vi "UI_page12.vi"(10 "传递队列输入":refnum<queue>, 11 "notifier":refnum<notifier>) -> ()   [LabVIEW 2012]
uses:
  <vilib>/Utility/miscctls.llb/LVDateTimeRec.ctl
  <vilib>/GPower/VIRegister/Library/Convert/ToBool.vi
  <vilib>/GPower/VIRegister/Library/Convert/ToU32.vi
  <vilib>/GPower/VIRegister/Library/Convert/ToU8.vi
  <vilib>/GPower/VIRegister/Library/SubVIs/FindRegisterData.vi
  <vilib>/GPower/VIRegister/Library/SubVIs/ReadSub.vi
  <vilib>/GPower/VIRegister/Library/SubVIs/WriteSub.vi
  <vilib>/GPower/Error/Library/FilterCodes.vi
  <vilib>/GPower/Error/Library/Filter/FilterMulti.vi
  <vilib>/GPower/VIRegister/Library/QManager/GetRegisterData.vi
  <vilib>/GPower/Error/Library/SetError.vi
  <vilib>/GPower/Error/Library/SplitAppended.vi
  <vilib>/GPower/VIRegister/Library/QManager/QManagerAction.vi
  <vilib>/GPower/Error/Library/ErrorType.vi
  <vilib>/GPower/Error/Library/SubVIs/ExplanationToError.vi
  <vilib>/GPower/VIRegister/Library/QManager/GetQName.vi
  <vilib>/GPower/VIRegister/Library/QManager/StartQManager.vi
  <vilib>/Utility/error.llb/Trim Whitespace.vi
  <vilib>/dlg_ctls.llb/Space Constant.vi
  <vilib>/Utility/error.llb/Error Code Database.vi
  <vilib>/GPower/Error/Library/SubVIs/SetStatus.vi
  <vilib>/GPower/Error/Library/AppendErrors.vi
  <vilib>/GPower/Error/Library/Append/AppendSingle.vi
  <vilib>/GPower/VIRegister/VIRegister.lvlib
  <vilib>/measure/NI_MABase.lvlib
panel:
  out "试验已用时":timestamp=timestamp(-28800 s since 1904-01-01) format="%<%H:%M:%S>T"
  in  "测试时间设定":timestamp=timestamp(-28800 s since 1904-01-01) format="%<%H:%M:%S>T"
  in  "停止测量":bool
  in  "开始测量":bool
  out "温度":string
  out "脉冲计数":string
  out "主份G3陀螺脉冲计数":dbl(graph)
  out "主份A3加速度计脉冲计数":dbl(graph)
  out "主份G2陀螺脉冲数":dbl(graph)
  out "主份A2加速度计脉冲计数":dbl(graph)
  out "主份G1陀螺脉冲数":dbl(graph)
  out "主份A1加速度计脉冲计数":dbl(graph)
  out "正确帧计数":u16
  out "错误帧计数":u32
  in  "加计大小量程":enum32{"小量程", "大量程"}(radio)=enum."大量程"
  in  "穿插错误":bool
  in  "少数据字":bool
  in  "少验和":bool
  in  "少帧头":bool
  in  "验和错":bool
  in  "帧头错":bool
  in  "无数据":bool
  in  "地检按钮":bool
  in  "加表频率":dbl=1.0 min=0.1 max=10.0 step=0.1
  in  "加表幅值":dbl=1.0
  in  "陀螺频率":dbl=1.0 min=0.1 max=10.0 step=0.1
  in  "陀螺幅值":dbl=1.0
  # "主  份"
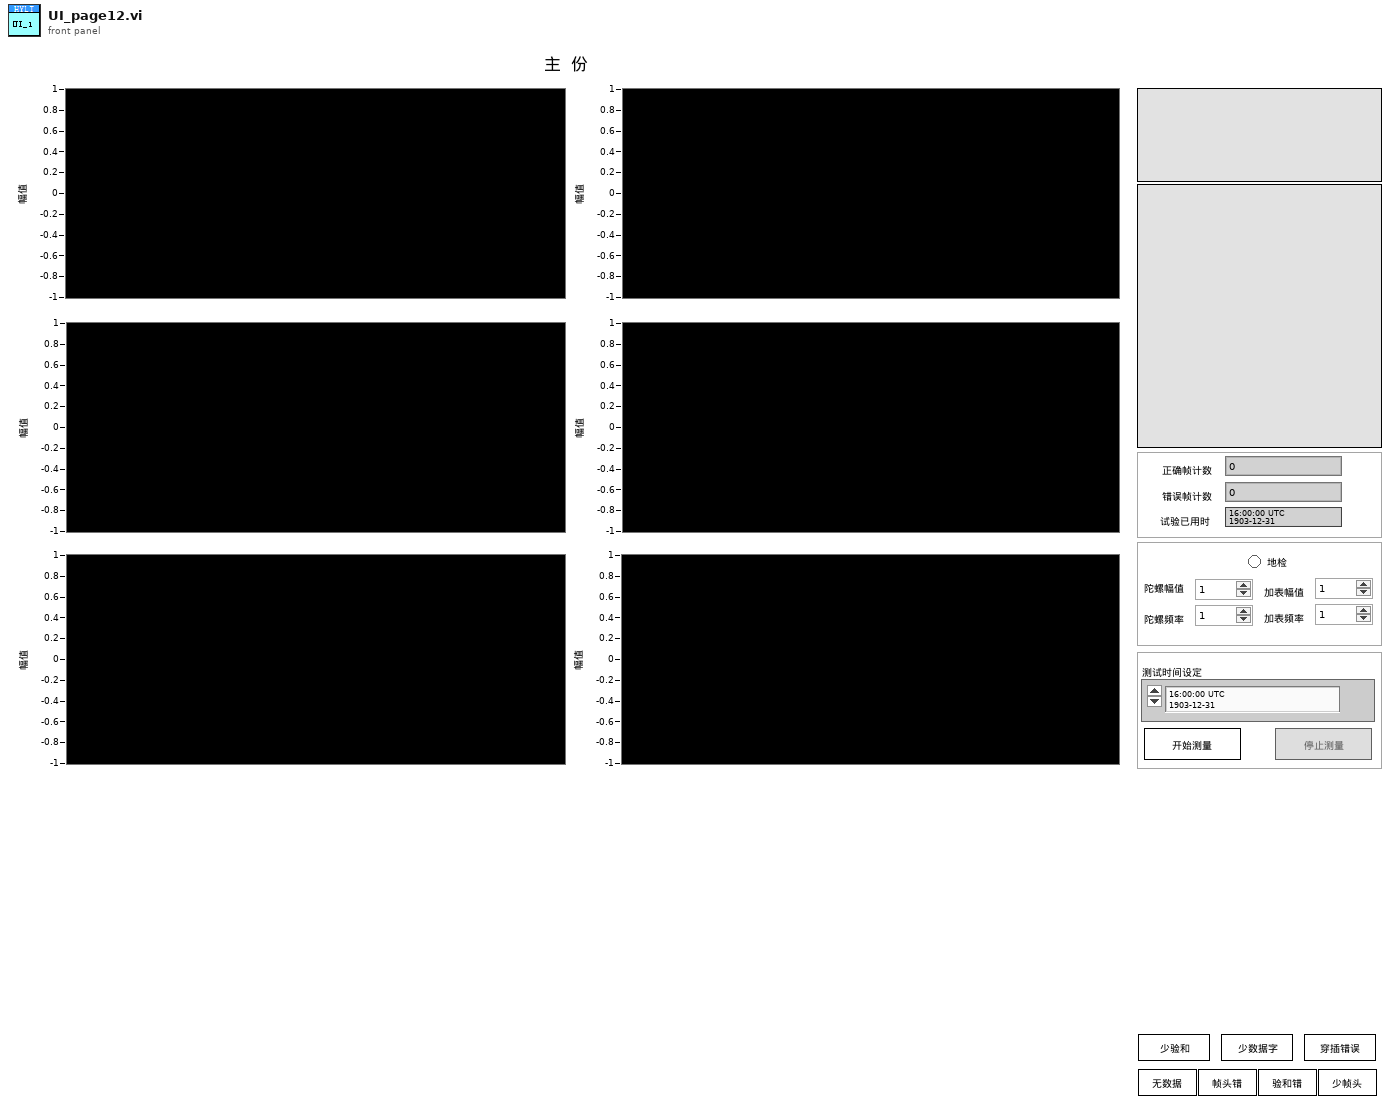
[diagram p1: front panel]
types:
  T1 = typedef "LVDateTimeRec.ctl" = cluster{"fractional second":dbl, "second":i32, "minute":i32, "hour":i32, "day of month":i32, "month":i32, "year":i32, "day of week":i32, "day of year":i32, "DST":i32}
  T2 = enum8{"Enabled", "Disabled", "Disabled and Grayed Out"}
  T3 = enum32{"invalid app kind", "Development System", "Run Time System", "Student Edition", "Embedded LabVIEW", "Evaluation", "Custom"}
  T4 = enum32{"Invalid", "Standard", "Closed", "Hidden", "Minimized", "Maximized"}
  T5 = cluster{"Core":cluster{"Current VI Reference":refnum<vi>, "Close Panel on Exit?":bool}, "传递队列输入":refnum<queue>, "信息帧":cluster{" 数据帧名称":string, " 数据":string, "备用操作符":bool, "起始地址":i32, "读写标志":i32, "长度":i32}, "主份控制指令":u16, "备份控制指令":u16, "notifier ":refnum<notifier>, "秒计数":i64, "起始时间":i64, "定时控制":bool}
  T6 = cluster{" 数据帧名称":string, " 数据":string, "备用操作符":bool, "起始地址":i32, "读写标志":i32, "长度":i32}
  T7 = cluster{"Current VI Reference":refnum<vi>, "Close Panel on Exit?":bool}
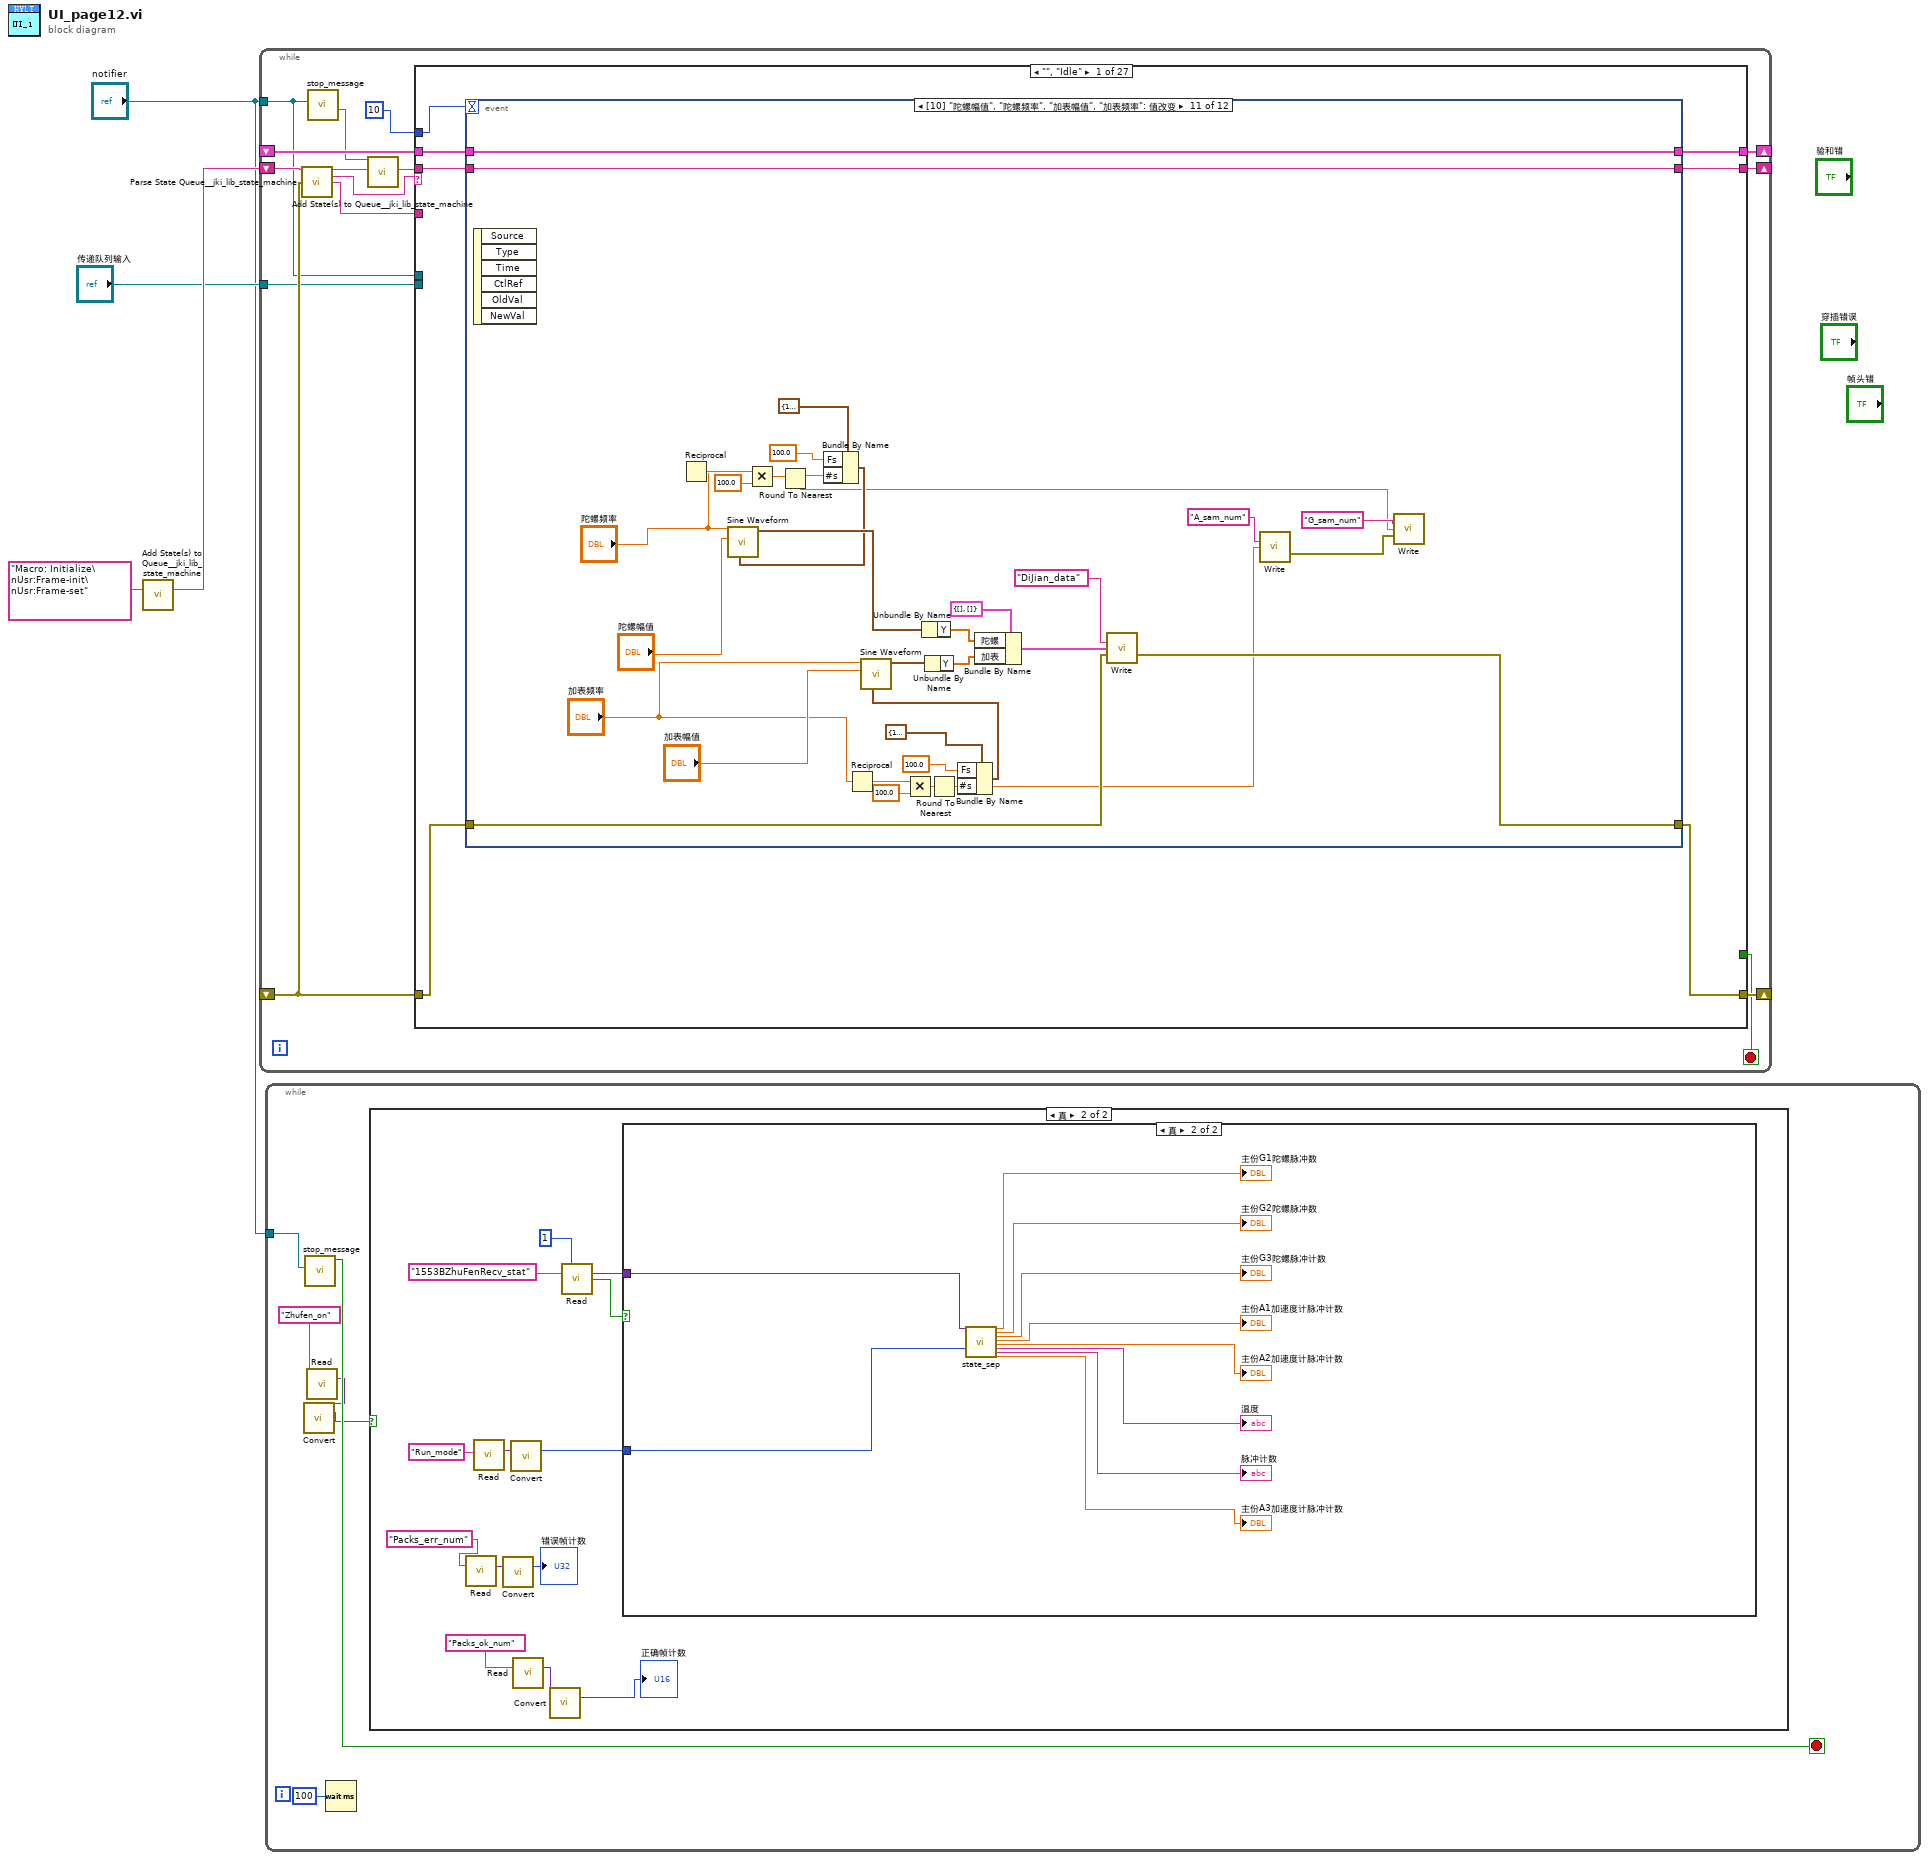
[diagram p0: block diagram]
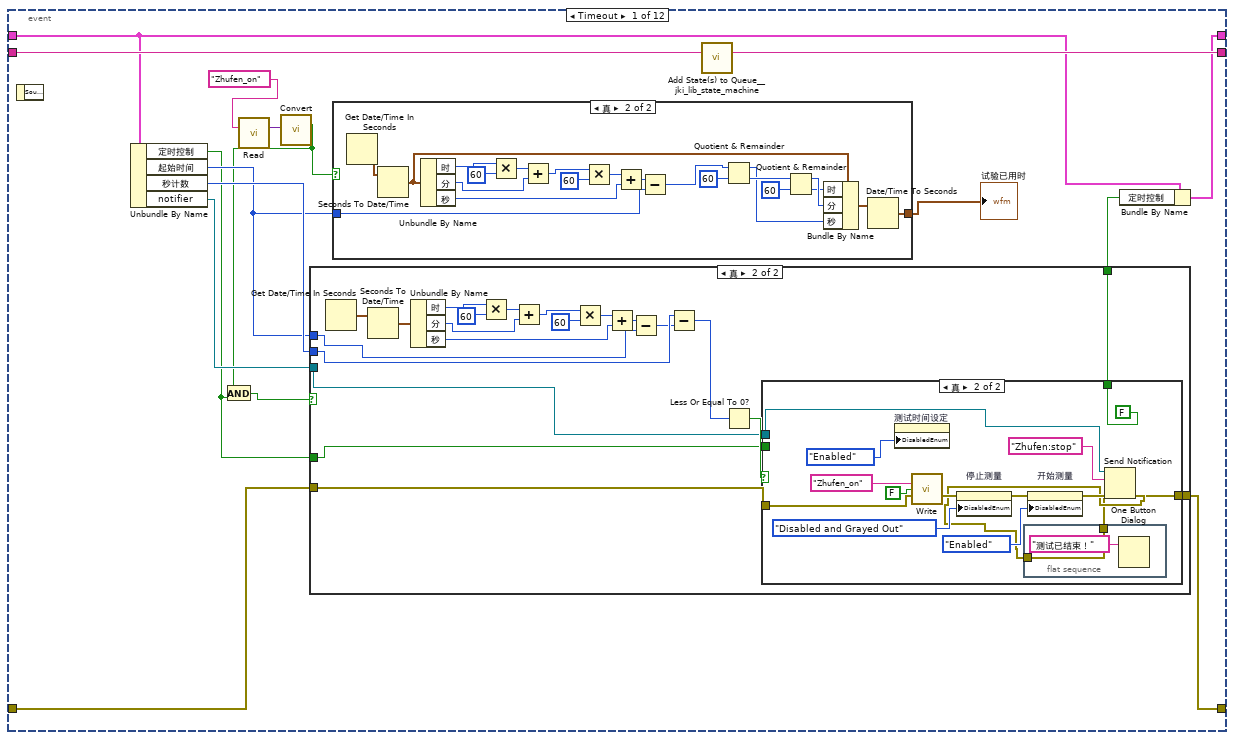
[diagram p4: hidden frame]
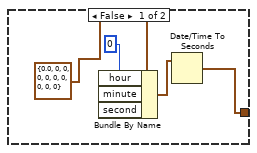
[diagram p5: hidden frame]
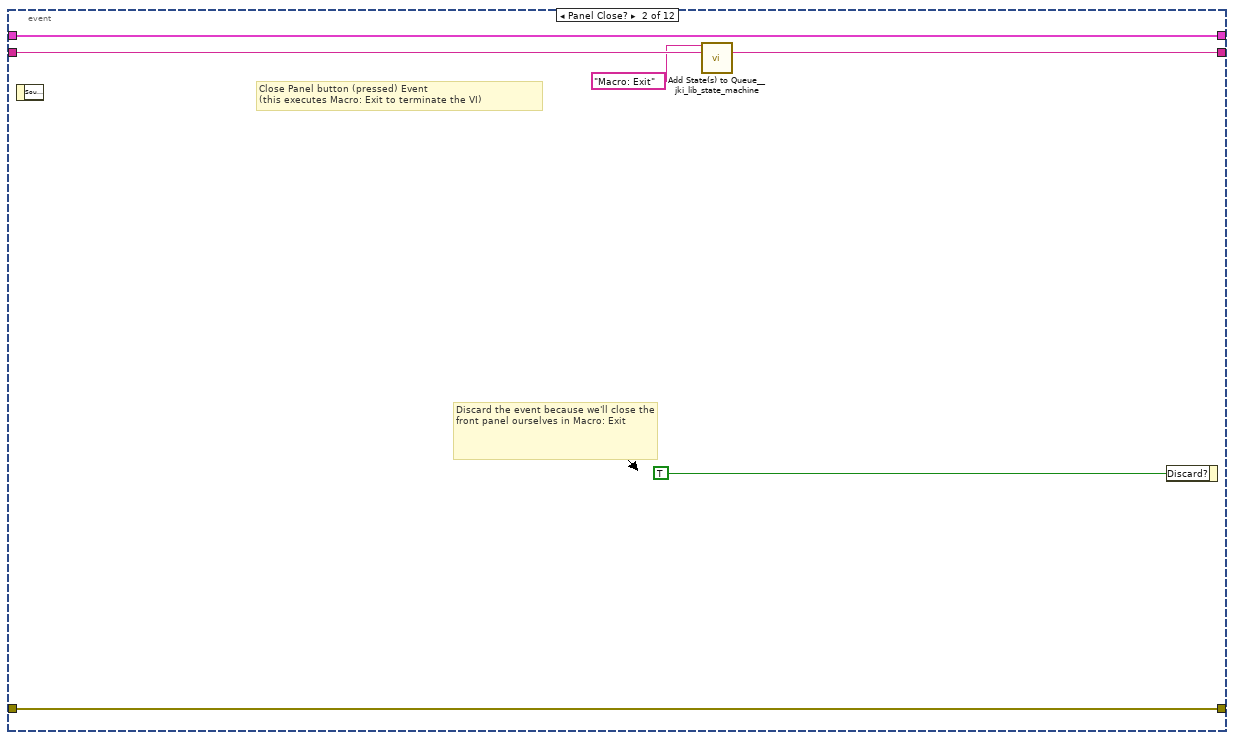
[diagram p8: hidden frame]
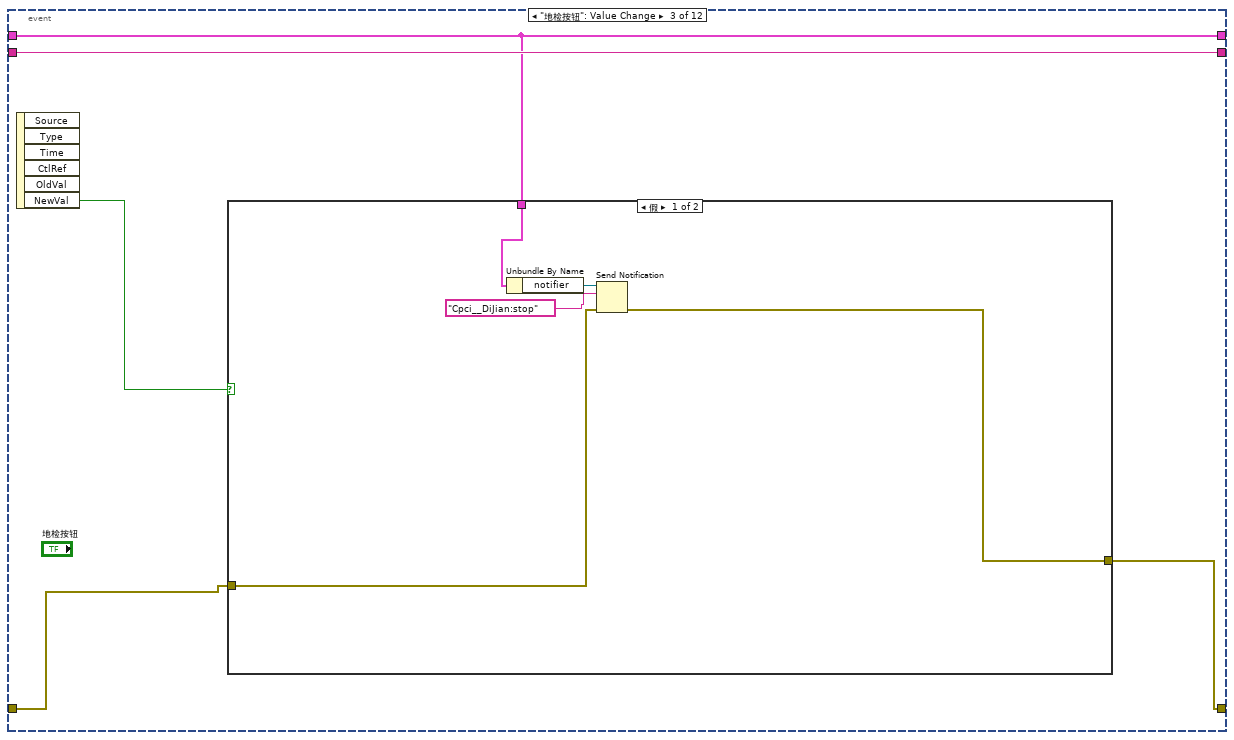
[diagram p9: hidden frame]
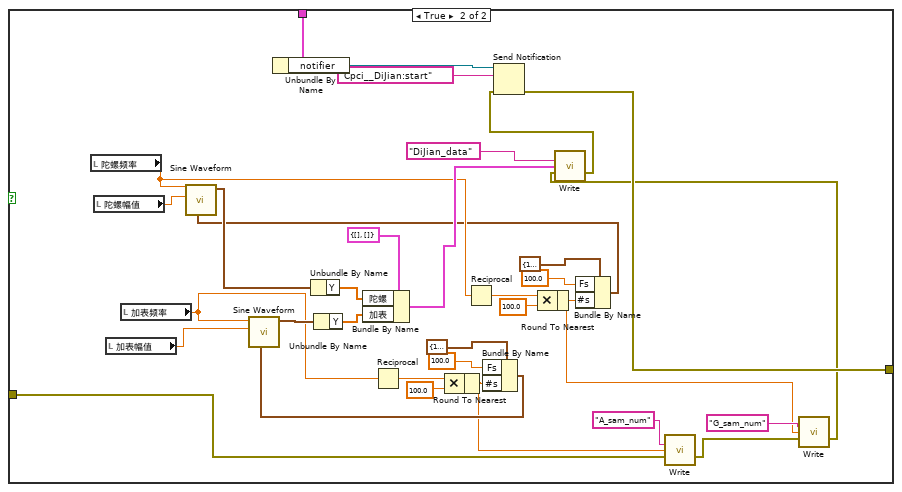
[diagram p10: hidden frame]
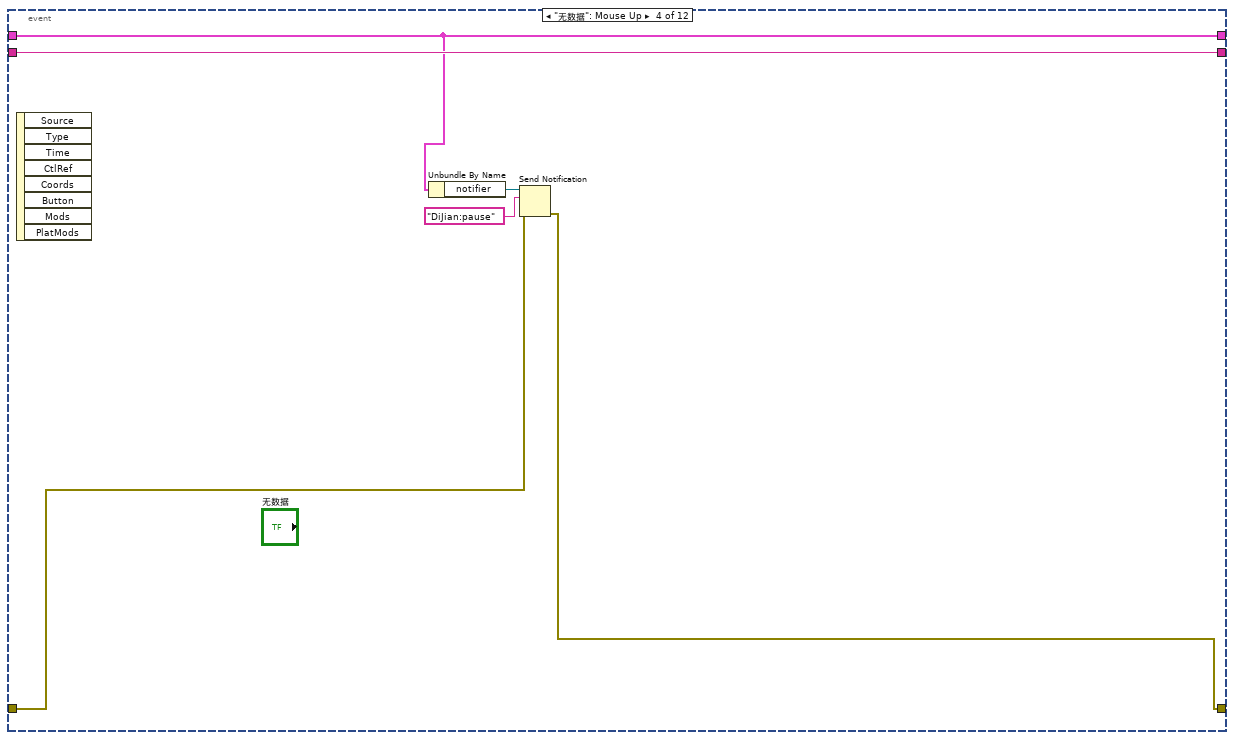
[diagram p11: hidden frame]
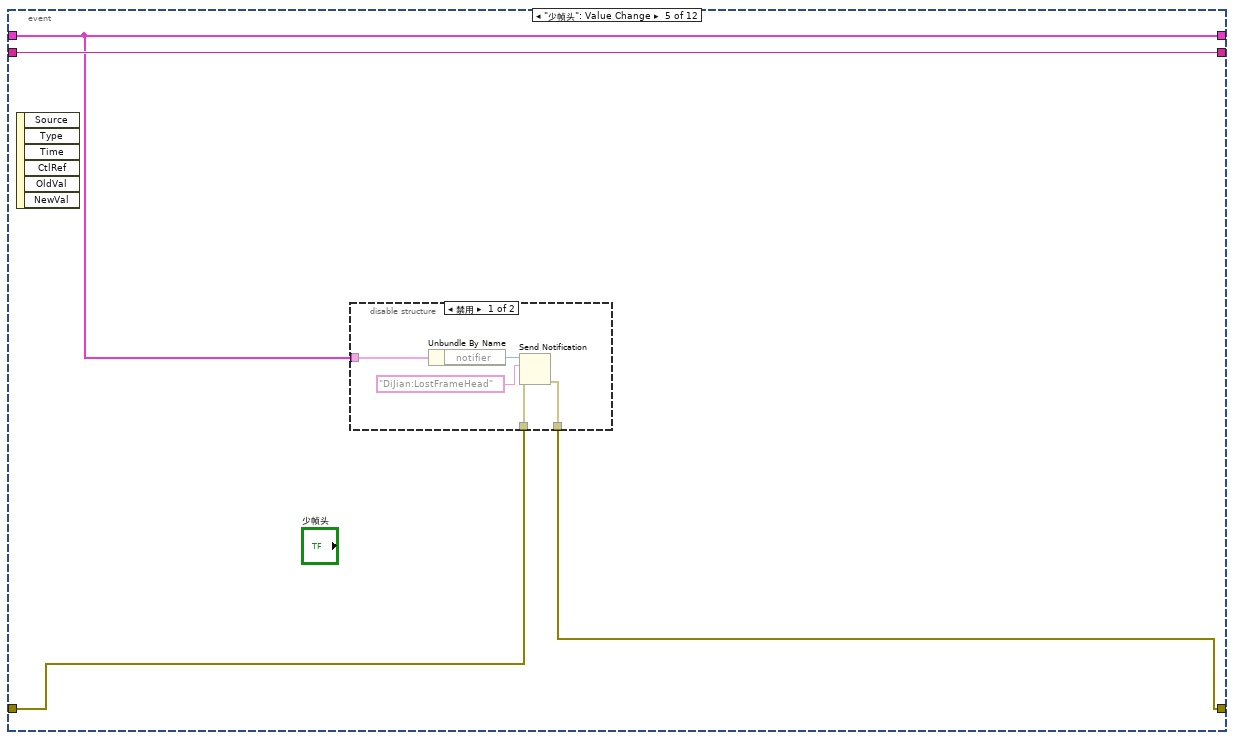
[diagram p12: hidden frame]
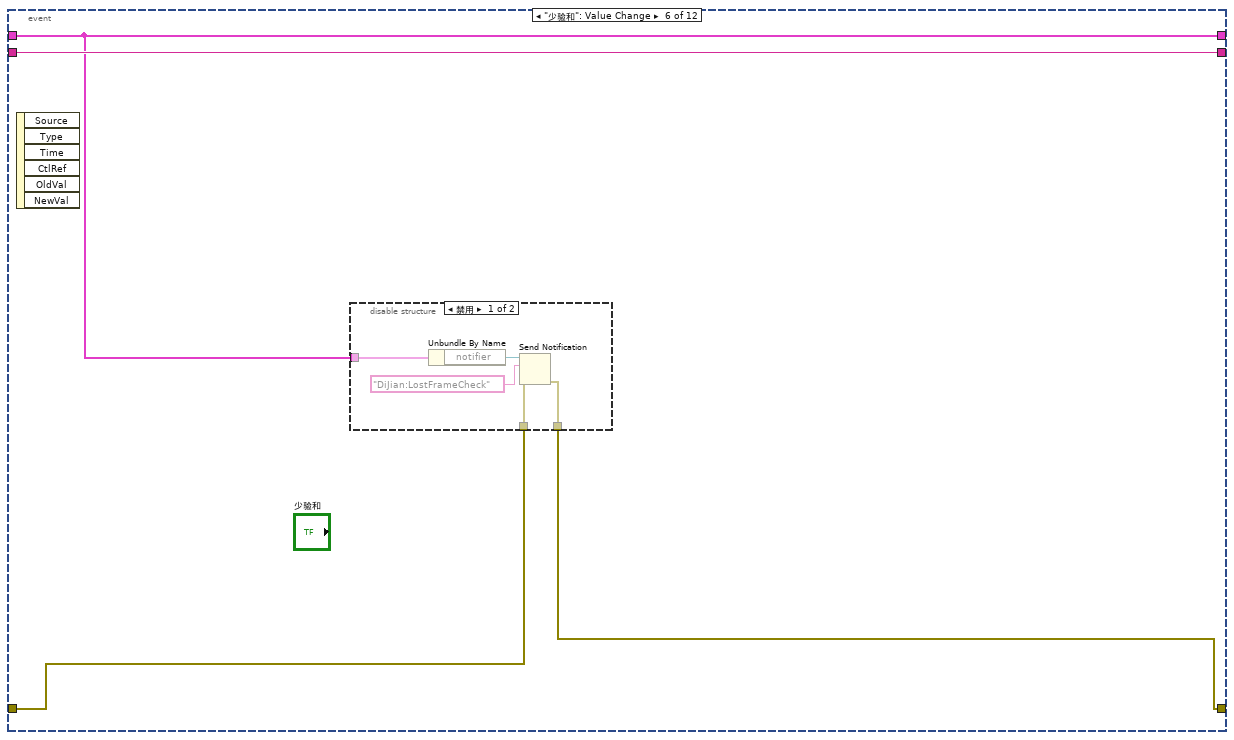
[diagram p14: hidden frame]
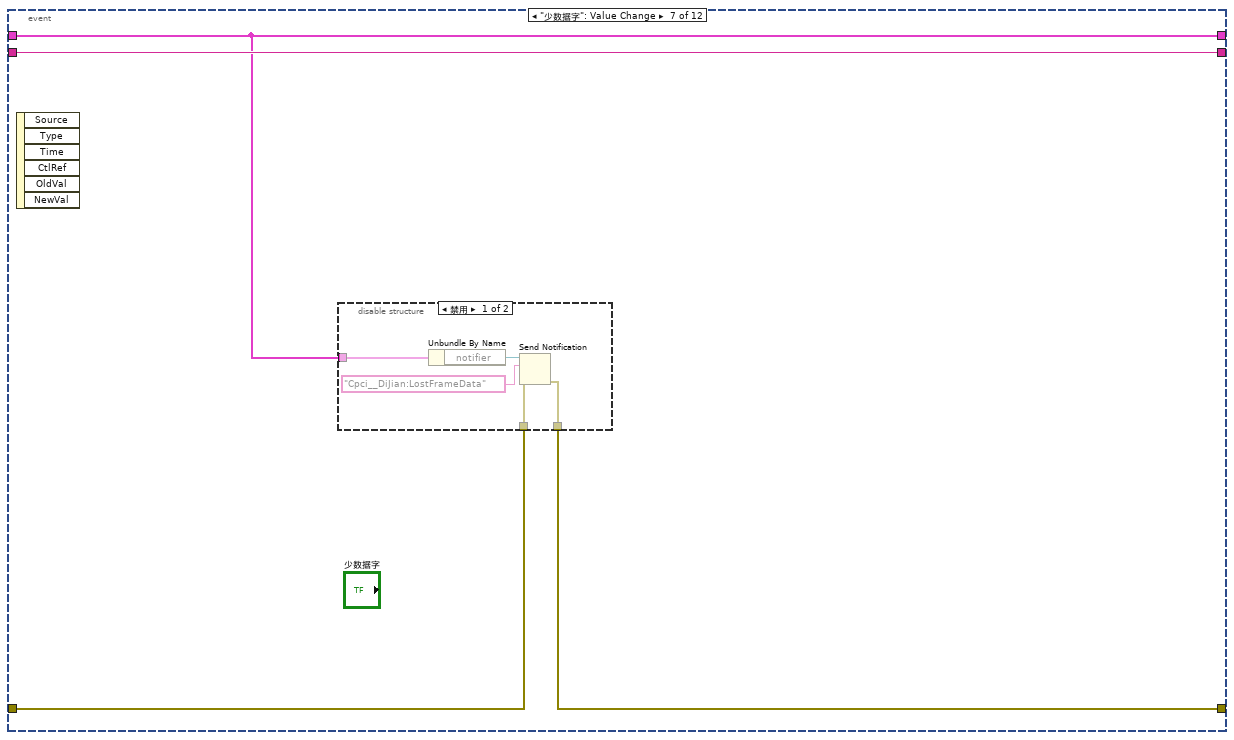
[diagram p16: hidden frame]
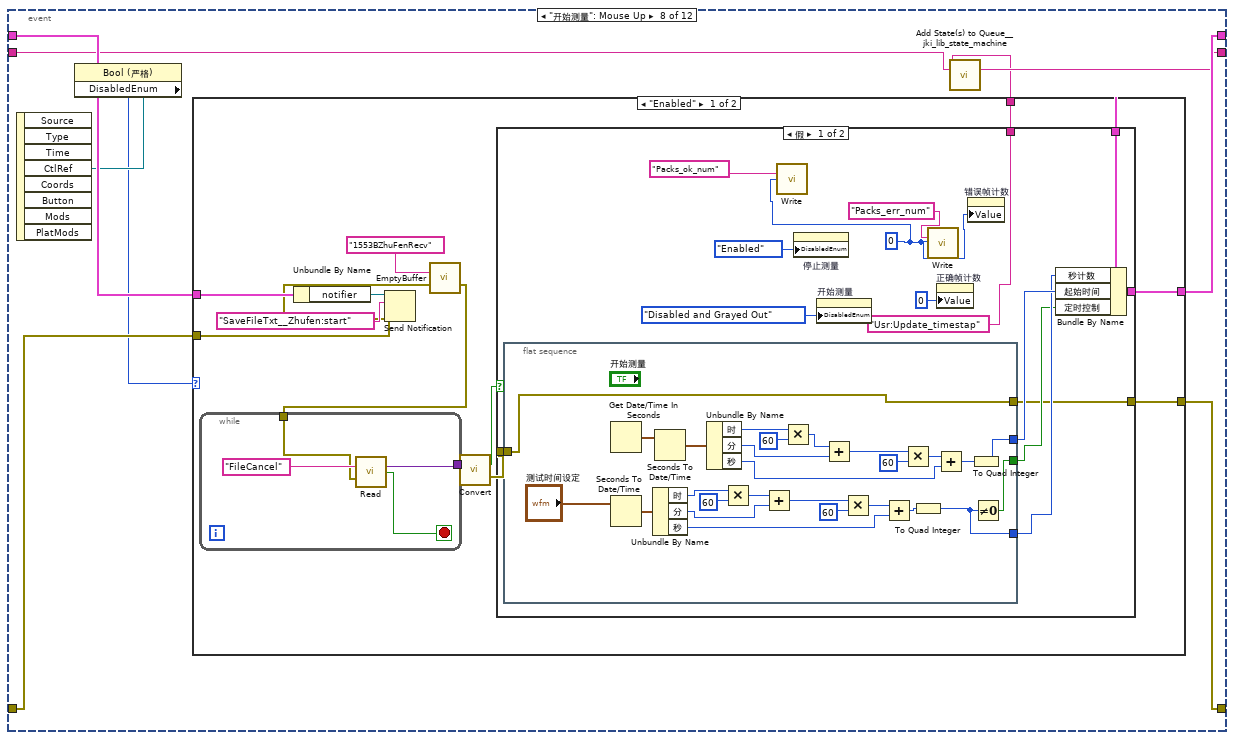
[diagram p18: hidden frame]
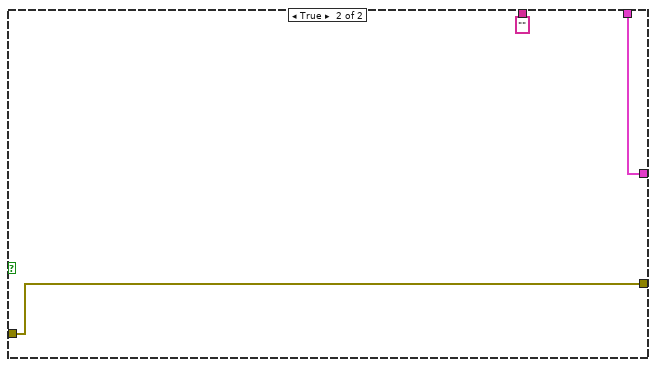
[diagram p19: hidden frame]
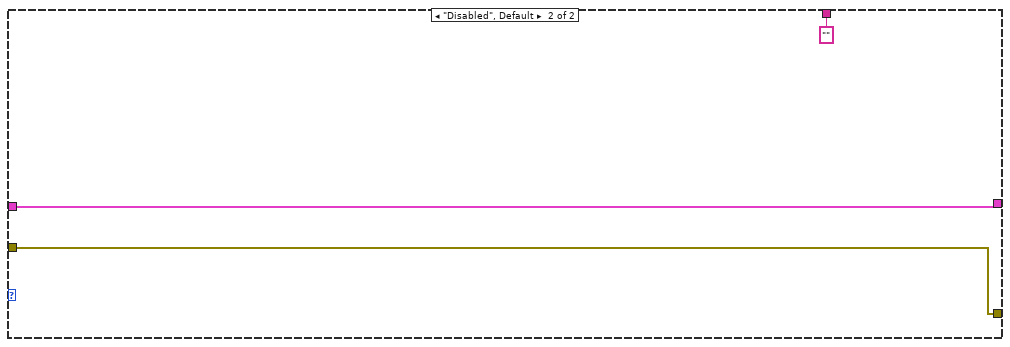
[diagram p20: hidden frame]
diagram:
  n1 = call <vilib>:"Add State(s) to Queue__jki_lib_state_machine.vi"("State(s) in (\"\")"="Macro: Initialize\nUsr:Frame-init\nUsr:Frame-set") -> ("States Out"=w4:string)  [unwired: 14 in]
  n2 = while "JKI - String-Based Queued State Machine (Basic) v1.0" {
    shift-right: [w13] -> _
    shift-left: _ -> [w12]
    shift-right: [w16] -> _
    shift-left: _ -> [w10]
    shift-right: [w15] -> _
    shift-left: w4 -> [w17]
    tunnel: "notifier" -> [w5]
    tunnel: "传递队列输入" -> [w6]
    stop <- w14 stop-if-true
    n3 = call <vilib>:"Parse State Queue__jki_lib_state_machine.vi"("State Queue"=w17, "Error In (no error)"=w10) -> ("Remaining States"=w9:string, "Current State"=w19:string, "Arguments"=w18:string)  [unwired: 11 in]
    n4 = call "stop_message.vi"("notifier"=w5) -> ("通知"=w8:string)  [unwired: 9 in, 1 out]
    n5 = call <vilib>:"Add State(s) to Queue__jki_lib_state_machine.vi"("State(s) in Front (\"\")"=w8, "State(s) in (\"\")"=w9) -> ("States Out"=w7:string)  [unwired: 13 in]
    n6 = case shown="\"\", \"Idle\"" w19 {
      selector: w19 -> [_ _ w352 _ _ _ _ _ _ _ _ _ _ _ _ _ _ _ _ _ _ _ _ _ _ _ _]
      tunnel: w7 -> [w20 w351 w356 w374 w380 w385 w389 w405 w411 w415 w424 w430 w440 w472 w477 w487 w491 w498 w518 w538 w557 w583 w599 w604 w609 w621 w639]
      tunnel: w18 -> [_ _ _ _ _ _ _ _ _ _ _ w425 w435 _ _ _ _ w492 w512 w532 _ _ _ _ _ _ _]
      tunnel: w12 -> [w25 w348 w354 w365 w377 w383 w386 _ w406 w412 w422 w428 w436 w469 w474 w484 w488 w496 w516 w536 w555 w581 w596 w601 w606 w617 w626]
      tunnel: [w24 w349 w358 w371 errorcluster {"status"=FALSE, "code"=0, "source"=""} ("error out") w382 w387 w402 w407 w413 w421 w426 w437 w470 w475 w485 w489 w494 w514 w534 w553 w579 w597 w602 w607 w619 w624] -> w16
      tunnel: w10 -> [w23 w349 w357 w371 w376 w382 w387 w402 w408 w413 w421 w427 w438 w470 w475 w485 w489 w495 w515 w535 w554 w580 w597 w602 w607 w619 w624]
      tunnel: [w26 w350 w355 w373 w379 w384 w388 w404 w410 w414 w423 w429 w439 w471 w476 w486 w490 w497 w517 w537 w556 w582 w598 w603 w608 w620 w638] -> w15
      tunnel: [_ _ _ _ _ TRUE _ _ _ _ _ _ _ _ _ _ _ _ _ _ _ _ _ _ _ _ _] -> w14
      tunnel: [w22 w348 w354 w372 w377 w383 w386 w403 w406 w412 w422 w428 w436 w469 w474 w484 w488 w493 w513 w533 w552 w578 w596 w601 w605 w617 w625] -> w13
      tunnel: 10 ("Timeout") -> [w21 _ _ _ _ _ _ _ _ _ _ _ _ _ _ _ _ _ _ _ _ _ _ _ _ _ _]
      tunnel: w6 -> [_ _ _ _ _ _ _ w399 _ _ _ _ _ _ _ _ _ _ _ _ _ _ _ _ _ _ _]
      tunnel: w5 -> [_ _ _ _ _ _ _ w395 _ _ _ _ _ _ _ _ _ _ _ _ _ _ _ _ _ _ _]
      frame "", "Idle" {
        n7 = event shown="[10] \"陀螺幅值\", \"陀螺频率\", \"加表幅值\", \"加表频率\": 值改变" {
          selector: _ -> [_ _ _ _ _ _ _ _ _ _ _ _]
          dyn-events: _ -> [_ _ _ _ _ _ _ _ _ _ _ _]
          timeout: w21 -> [_ _ _ _ _ _ _ _ _ _ _ _]
          tunnel: w20 -> [w42 w114 w119 w165 w169 w178 w187 w195 w271 w306 w337 w339]
          tunnel: [w41 w113 w119 w165 w169 w178 w187 w194 w271 w306 w337 w339] -> w26
          tunnel: w25 -> [w36 w111 w118 w164 w168 w177 w186 w200 w268 w293 w338 w340]
          tunnel: [w37 w112 w116 w162 w166 w175 w184 w198 w269 w305 w334 w341] -> w24
          tunnel: w23 -> [w38 w112 w117 w163 w167 w176 w185 w201 w270 w305 w333 w342]
          tunnel: [w35 w111 w118 w164 w168 w177 w186 w199 w267 w292 w338 w340] -> w22
          event Timeout {
            n8 = event-data() -> ()  [unwired: 1 in, 1 out]
            n9 = Unbundle By Name(w36) -> ("定时控制"=w27:bool, "起始时间"=w33:i64, "秒计数"=w40:i64, "notifier"=w39:refnum<notifier>)
            n10 = call <vilib>:"Read.vi"("Register name"="Zhufen_on") -> ("Register value"=w30:variant)  [unwired: 11 in, 3 out]
            n11 = call-poly <vilib>:"Convert.vi"("Register value in"=w30) -> ("Register value out"=w29:bool)  [unwired: 13 in, 1 out]
            n12 = And(x=w29, y=w27) -> (x .and. y?=w28:bool)
            n13 = case shown="真" w28 {
              tunnel: w33 -> [_ w81]
              tunnel: w40 -> [_ w80]
              tunnel: w39 -> [_ w74]
              tunnel: w38 -> [w69 w73]
              tunnel: [w69 w72] -> w37
              tunnel: [w68 w71] -> w34
              tunnel: w27 -> [w68 w70]
              frame False {
              }
              frame True {
                n14 = Get Date/Time In Seconds() -> (seconds since 1Jan1904=w77:timestamp)
                n15 = Seconds To Date/Time(time stamp (now)=w77) -> (date time rec=w78:T1)  [unwired: 1 in]
                n16 = Unbundle By Name(w78) -> ("时"=w83:i32, "分"=w86:i32, "秒"=w90:i32)
                n17 = Multiply(x=w83, y=60) -> (x*y=w85:i32)
                n18 = Add(x=w85, y=w86) -> (x+y=w87:i32)
                n19 = Multiply(x=w87, y=60) -> (x*y=w89:i32)
                n20 = Add(x=w89, y=w90) -> (x+y=w82:i32)
                n21 = Subtract(x=w82, y=w81) -> (x-y=w79:i64)
                n22 = Subtract(x=w80, y=w79) -> (x-y=w76:i64)
                n23 = Less Or Equal To 0?(x=w76) -> (x <= 0?=w75:bool)
                n24 = case shown="真" w75 {
                  tunnel: w74 -> [_ w98]
                  tunnel: w73 -> [w92 w97]
                  tunnel: [w92 w93] -> w72
                  tunnel: [w91 FALSE] -> w71
                  tunnel: w70 -> [w91 _]
                  frame False {
                  }
                  frame True {
                    n25 = property on="测试时间设定" class="AbsTime (严格)"("DisabledEnum"=T2."Enabled" ("禁用")) -> ()  [unwired: 2 in, 2 out]
                    n26 = call <vilib>:"Write.vi"("Register name"="Zhufen_on", "Register value"=FALSE ("停止测量"), "Error in"=w97) -> ("Error out"=w100:errorcluster)  [unwired: 10 in, 2 out]
                    n27 = property on="停止测量" class="Bool (严格)"(error in=w100, "DisabledEnum"=T2."Disabled and Grayed Out" ("禁用")) -> (error out=w101:errorcluster)  [unwired: 1 in, 1 out]
                    n28 = flat-sequence {
                      tunnel: w94 -> [w107]
                      tunnel: [w107] -> w93
                      frame #0 {
                        n29 = One Button Dialog(message="测试已结束！" ("消息")) -> ()  [unwired: 1 in, 1 out]
                      }
                    }
                    n30 = property on="开始测量" class="Bool (严格)"(error in=w101, "DisabledEnum"=T2."Enabled" ("禁用")) -> (error out=w99:errorcluster)  [unwired: 1 in, 1 out]
                    n31 = Send Notification(notification="Zhufen:stop" ("通知"), notifier=w98, error in (no error)=w99) -> (error out=w94:errorcluster)  [unwired: 1 out]
                  }
                }
              }
            }
            n32 = case shown="真" w29 {
              tunnel: w33 -> [_ w57]
              tunnel: [w43 w49] -> w32
              frame False {
                w45 = 0 ("时")
                n33 = Bundle By Name(cluster=T1 {"fractional second"=0.0, "second"=0, "minute"=0, "hour"=0, "day of month"=0, "month"=0, "year"=0, "day of week"=0, "day of year"=0, "DST"=0} ("日期时间记录 2"), "hour"=w45, "minute"=w45, "second"=w45) -> (w46:T1)
                n34 = Date/Time To Seconds(2:w46) -> (0:w43:timestamp)  [unwired: 1 in]
              }
              frame True {
                n35 = Get Date/Time In Seconds() -> (seconds since 1Jan1904=w67:timestamp)
                n36 = Seconds To Date/Time(time stamp (now)=w67) -> (date time rec=w50:T1)  [unwired: 1 in]
                n37 = Unbundle By Name(w50) -> ("时"=w65:i32, "分"=w62:i32, "秒"=w58:i32)
                n38 = Multiply(x=w65, y=60) -> (x*y=w63:i32)
                n39 = Add(x=w63, y=w62) -> (x+y=w61:i32)
                n40 = Multiply(x=w61, y=60) -> (x*y=w59:i32)
                n41 = Add(x=w59, y=w58) -> (x+y=w66:i32)
                n42 = Subtract(x=w66, y=w57) -> (x-y=w47:i64)
                n43 = Quotient & Remainder(x=w47, y=60) -> (x-y*floor(x/y)=w48:i64, floor(x/y)=w52:i64)
                n44 = Quotient & Remainder(x=w52, y=60) -> (x-y*floor(x/y)=w55:i64, floor(x/y)=w54:i64)
                n45 = Bundle By Name(cluster=w50, "时"=w54, "分"=w55, "秒"=w48) -> (w56:T1)
                n46 = Date/Time To Seconds(2:w56) -> (0:w49:timestamp)  [unwired: 1 in]
              }
            }
            "试验已用时" <- w32
            n47 = call <vilib>:"Add State(s) to Queue__jki_lib_state_machine.vi"("State(s) in (\"\")"=w42) -> ("States Out"=w41:string)  [unwired: 14 in]
            n48 = Bundle By Name(cluster=w36, "定时控制"=w34) -> (w35:T5)
          }
          event Panel Close? {
            # "Discard the event because we'll close the front panel ourselves in Macro: Exit"
            # "Close Panel button (pressed) Event\n(this executes Macro: Exit to terminate the VI)"
            n49 = event-data() -> ()  [unwired: 1 in, 1 out]
            n50 = call <vilib>:"Add State(s) to Queue__jki_lib_state_machine.vi"("State(s) in Front (\"\")"="Macro: Exit", "State(s) in (\"\")"=w114) -> ("States Out"=w113:string)  [unwired: 13 in]
            n51 = event-data("Discard?"=TRUE) -> ()  [unwired: 1 in, 1 out]
          }
          event "地检按钮": Value Change {
            n52 = event-data() -> ("NewVal"=w115:bool)  [unwired: 1 in, 5 out]
            n53 = case shown="假" w115 {
              tunnel: [w120 w146] -> w116
              tunnel: w118 -> [w122 w156]
              tunnel: w117 -> [w121 w126]
              frame False {
                n54 = Unbundle By Name(w122) -> ("notifier"=w123:refnum<notifier>)
                n55 = Send Notification(notification="Cpci__DiJian:stop" ("通知"), notifier=w123, error in (no error)=w121) -> (error out=w120:errorcluster)  [unwired: 1 out]
              }
              frame True {
                n56 = local read "陀螺频率"() -> (w135:dbl)
                n57 = local read "陀螺幅值"() -> (w148:dbl)
                n58 = local read "加表幅值"() -> (w149:dbl)
                n59 = local read "加表频率"() -> (w141:dbl)
                n60 = Unbundle By Name(w156) -> ("notifier"=w157:refnum<notifier>)
                n61 = Reciprocal(x=w141) -> (1/x=w145:dbl)
                n62 = Multiply(x=w145, y=100.0) -> (x*y=w132:dbl)
                n63 = Round To Nearest(number=w132) -> (nearest integer value=w127:dbl)
                n64 = Reciprocal(x=w135) -> (1/x=w139:dbl)
                n65 = Bundle By Name(cluster=cluster{"Fs":dbl, "#s":dbl} {"Fs"=1000.0, "#s"=1000.0} ("sampling info"), "Fs"=100.0, "#s"=w127) -> (w140:cluster{"Fs":dbl, "#s":dbl})
                n66 = call <vilib>:"Sine Waveform.vi"("sampling info"=w140, "amplitude"=w149, "frequency"=w141) -> ("signal out"=w153:waveform(dbl))  [unwired: 7 in, 1 out]
                n67 = Unbundle By Name(w153) -> ("Y"=w151:dbl[])
                n68 = Multiply(x=w139, y=100.0) -> (x*y=w130:dbl)
                n69 = Round To Nearest(number=w130) -> (nearest integer value=w128:dbl)
                n70 = Bundle By Name(cluster=cluster{"Fs":dbl, "#s":dbl} {"Fs"=1000.0, "#s"=1000.0} ("sampling info"), "Fs"=100.0, "#s"=w128) -> (w134:cluster{"Fs":dbl, "#s":dbl})
                n71 = call <vilib>:"Sine Waveform.vi"("sampling info"=w134, "amplitude"=w148, "frequency"=w135) -> ("signal out"=w154:waveform(dbl))  [unwired: 7 in, 1 out]
                n72 = Unbundle By Name(w154) -> ("Y"=w150:dbl[])
                n73 = Bundle By Name(cluster=cluster{"陀螺":dbl[], "加表":dbl[]} {"陀螺"=[], "加表"=[]} ("输入簇"), "陀螺"=w150, "加表"=w151) -> (w155:cluster{"陀螺":dbl[], "加表":dbl[]})
                n74 = call <vilib>:"Write.vi"("Register name"="A_sam_num", "Register value"=w127, "Error in"=w126) -> ("Error out"=w129:errorcluster)  [unwired: 10 in, 2 out]
                n75 = call <vilib>:"Write.vi"("Register name"="G_sam_num", "Register value"=w128, "Error in"=w129) -> ("Error out"=w125:errorcluster)  [unwired: 10 in, 2 out]
                n76 = call <vilib>:"Write.vi"("Register name"="DiJian_data", "Register value"=w155, "Error in"=w125) -> ("Error out"=w147:errorcluster)  [unwired: 10 in, 2 out]
                n77 = Send Notification(notification="Cpci__DiJian:start" ("通知"), notifier=w157, error in (no error)=w147) -> (error out=w146:errorcluster)  [unwired: 1 out]
              }
            }
          }
          event "无数据": Mouse Up {
            n78 = event-data() -> ()  [unwired: 1 in, 8 out]
            n79 = Unbundle By Name(w164) -> ("notifier"=w160:refnum<notifier>)
            n80 = Send Notification(notification="DiJian:pause" ("通知"), notifier=w160, error in (no error)=w163) -> (error out=w162:errorcluster)  [unwired: 1 out]
          }
          event "少帧头": Value Change {
            n81 = event-data() -> ()  [unwired: 1 in, 6 out]
            n82 = disable-structure shown="禁用" {
              disable-tunnel: w168 -> [w174 _]
              disable-tunnel: w167 -> [w173 _]
              disable-tunnel: [w172 _] -> w166
              frame Disabled {
                n83 = Unbundle By Name(w174) -> ("notifier"=w170:refnum<notifier>)
                n84 = Send Notification(notification="DiJian:LostFrameHead" ("通知"), notifier=w170, error in (no error)=w173) -> (error out=w172:errorcluster)  [unwired: 1 out]
              }
              frame Enabled {
              }
            }
          }
          event "少验和": Value Change {
            n85 = event-data() -> ()  [unwired: 1 in, 6 out]
            n86 = disable-structure shown="禁用" {
              disable-tunnel: w177 -> [w183 _]
              disable-tunnel: w176 -> [w182 _]
              disable-tunnel: [w181 _] -> w175
              frame Disabled {
                n87 = Unbundle By Name(w183) -> ("notifier"=w179:refnum<notifier>)
                n88 = Send Notification(notification="DiJian:LostFrameCheck" ("通知"), notifier=w179, error in (no error)=w182) -> (error out=w181:errorcluster)  [unwired: 1 out]
              }
              frame Enabled {
              }
            }
          }
          event "少数据字": Value Change {
            n89 = event-data() -> ()  [unwired: 1 in, 6 out]
            n90 = disable-structure shown="禁用" {
              disable-tunnel: w186 -> [w192 _]
              disable-tunnel: w185 -> [w191 _]
              disable-tunnel: [w190 _] -> w184
              frame Disabled {
                n91 = Unbundle By Name(w192) -> ("notifier"=w188:refnum<notifier>)
                n92 = Send Notification(notification="Cpci__DiJian:LostFrameData" ("通知"), notifier=w188, error in (no error)=w191) -> (error out=w190:errorcluster)  [unwired: 1 out]
              }
              frame Enabled {
              }
            }
          }
          event "开始测量": Mouse Up {
            n93 = event-data() -> ("CtlRef"=w197:refnum<vi>)  [unwired: 1 in, 7 out]
            n94 = property class="Bool (严格)"(reference=w197) -> ("DisabledEnum"=w196:T2)  [unwired: 1 in, 2 out]
            n95 = case shown="\"Enabled\"" w196 {
              tunnel: w201 -> [w212 w263]
              tunnel: w200 -> [w211 w264]
              tunnel: [w210 w264] -> w199
              tunnel: [w209 w263] -> w198
              tunnel: [w202 "" ("State(s) in Front (\"\")")] -> w193
              frame "Enabled" {
                n96 = Unbundle By Name(w211) -> ("notifier"=w213:refnum<notifier>)
                n97 = Send Notification(notification="SaveFileTxt__Zhufen:start" ("通知"), notifier=w213, error in (no error)=w212) -> (error out=w205:errorcluster)  [unwired: 1 out]
                n98 = call <vilib>:"EmptyBuffer.vi"("Register name"="1553BZhuFenRecv", "Error in"=w205) -> ("Error out"=w204:errorcluster)  [unwired: 11 in, 2 out]
                n99 = while {
                  tunnel: w204 -> [w260]
                  tunnel: [w258] -> w208
                  stop <- w259 stop-if-true
                  n100 = call <vilib>:"Read.vi"("Register name"="FileCancel", "Error in"=w260) -> ("Register value"=w258:variant, "Register value read?"=w259:bool)  [unwired: 10 in, 2 out]
                }
                n101 = call-poly <vilib>:"Convert.vi"("Register value in"=w208) -> ("Register value out"=w206:bool, "Error out"=w207:errorcluster)  [unwired: 13 in]
                n102 = case shown="假" w206 {
                  tunnel: w211 -> [w226 w256]
                  tunnel: [w223 w256] -> w210
                  tunnel: [w221 w257] -> w209
                  tunnel: w207 -> [w220 w257]
                  tunnel: ["Usr:Update_timestap" ("State(s) in Front (\"\")") "" ("State(s) in Front (\"\")")] -> w202
                  frame False {
                    w217 = u32 0
                    n103 = flat-sequence {
                      tunnel: [w232] -> w225
                      tunnel: [w231] -> w224
                      tunnel: [w230] -> w222
                      tunnel: w220 -> [w229]
                      tunnel: [w229] -> w221
                      frame #0 {
                        n104 = Get Date/Time In Seconds() -> (seconds since 1Jan1904=w244:timestamp)
                        n105 = Seconds To Date/Time(time stamp (now)="测试时间设定") -> (date time rec=w253:T1)  [unwired: 1 in]
                        n106 = Unbundle By Name(w253) -> ("时"=w252:i32, "分"=w249:i32, "秒"=w245:i32)
                        n107 = Seconds To Date/Time(time stamp (now)=w244) -> (date time rec=w235:T1)  [unwired: 1 in]
                        n108 = Unbundle By Name(w235) -> ("时"=w236:i32, "分"=w239:i32, "秒"=w243:i32)
                        n109 = Multiply(x=w252, y=60) -> (x*y=w250:i32)
                        n110 = Add(x=w250, y=w249) -> (x+y=w248:i32)
                        n111 = Multiply(x=w236, y=60) -> (x*y=w238:i32)
                        n112 = Add(x=w238, y=w239) -> (x+y=w240:i32)
                        n113 = Multiply(x=w248, y=60) -> (x*y=w246:i32)
                        n114 = Add(x=w246, y=w245) -> (x+y=w233:i32)
                        n115 = Multiply(x=w240, y=60) -> (x*y=w242:i32)
                        n116 = To Quad Integer(1:w233) -> (0:w231:i64)
                        n117 = Add(x=w242, y=w243) -> (x+y=w234:i32)
                        n118 = To Quad Integer(1:w234) -> (0:w232:i64)
                        n119 = Not Equal To 0?(x=w231) -> (x != 0?=w230:bool)
                      }
                    }
                    n120 = call <vilib>:"Write.vi"("Register name"="Packs_ok_num", "Register value"=w217) -> ()  [unwired: 11 in, 3 out]
                    n121 = property on="停止测量" class="Bool (严格)"("DisabledEnum"=T2."Enabled" ("禁用")) -> ()  [unwired: 2 in, 2 out]
                    n122 = property on="开始测量" class="Bool (严格)"("DisabledEnum"=T2."Disabled and Grayed Out" ("禁用")) -> ()  [unwired: 2 in, 2 out]
                    n123 = call <vilib>:"Write.vi"("Register name"="Packs_err_num", "Register value"=w217) -> ()  [unwired: 11 in, 3 out]
                    n124 = property on="正确帧计数" class="DigNum (严格)"("Value"=u16 0 ("脉冲  累计")) -> ()  [unwired: 2 in, 2 out]
                    n125 = property on="错误帧计数" class="DigNum (严格)"("Value"=w217) -> ()  [unwired: 2 in, 2 out]
                    n126 = Bundle By Name(cluster=w226, "秒计数"=w224, "起始时间"=w225, "定时控制"=w222) -> (w223:T5)
                  }
                  frame True {
                  }
                }
              }
              frame "Disabled", Default {
              }
            }
            n127 = call <vilib>:"Add State(s) to Queue__jki_lib_state_machine.vi"("State(s) in Front (\"\")"=w193, "State(s) in (\"\")"=w195) -> ("States Out"=w194:string)  [unwired: 13 in]
          }
          event "停止测量": Mouse Up {
            n128 = event-data() -> ("CtlRef"=w266:refnum<vi>)  [unwired: 1 in, 7 out]
            n129 = property class="Bool (严格)"(reference=w266) -> ("DisabledEnum"=w265:T2)  [unwired: 1 in, 2 out]
            n130 = case shown="\"Enabled\"" w265 {
              tunnel: w270 -> [w279 w289]
              tunnel: [w278 w289] -> w269
              tunnel: w268 -> [w276 w288]
              tunnel: [w275 w288] -> w267
              frame "Enabled" {
                n131 = call <vilib>:"Write.vi"("Register name"="Zhufen_on", "Register value"=FALSE ("停止测量"), "Error in"=w279) -> ("Error out"=w280:errorcluster)  [unwired: 10 in, 2 out]
                n132 = property on="停止测量" class="Bool (严格)"(error in=w280, "DisabledEnum"=T2."Disabled and Grayed Out" ("禁用")) -> (error out=w281:errorcluster)  [unwired: 1 in, 1 out]
                n133 = property on="开始测量" class="Bool (严格)"(error in=w281, "DisabledEnum"=T2."Enabled" ("禁用")) -> (error out=w273:errorcluster)  [unwired: 1 in, 1 out]
                n134 = Unbundle By Name(w276) -> ("notifier"=w285:refnum<notifier>)
                n135 = property on="测试时间设定" class="AbsTime (严格)"(error in=w273, "DisabledEnum"=T2."Enabled" ("禁用")) -> (error out=w272:errorcluster)  [unwired: 1 in, 1 out]
                n136 = Send Notification(notification="Cpci__Zhufen:stop" ("通知"), notifier=w285, error in (no error)=w272) -> (error out=w278:errorcluster)  [unwired: 1 out]
                n137 = Bundle By Name(cluster=w276, "定时控制"=FALSE) -> (w275:T5)
              }
              frame "Disabled", Default {
              }
            }
          }
          event "测试时间设定": Value Change {
            n138 = event-data() -> ("NewVal"=w295:timestamp)  [unwired: 1 in, 5 out]
            n139 = Seconds To Date/Time(time stamp (now)=w295) -> (date time rec=w304:T1)  [unwired: 1 in]
            n140 = Unbundle By Name(w304) -> ("时"=w303:i32, "分"=w300:i32, "秒"=w296:i32)
            n141 = Multiply(x=w303, y=60) -> (x*y=w301:i32)
            n142 = Add(x=w301, y=w300) -> (x+y=w299:i32)
            n143 = Multiply(x=w299, y=60) -> (x*y=w297:i32)
            n144 = Add(x=w297, y=w296) -> (x+y=w291:i32)
            n145 = To Quad Integer(1:w291) -> (0:w294:i64)
            n146 = Not Equal To 0?(x=w291) -> (x != 0?=w290:bool)
            n147 = Bundle By Name(cluster=w293, "秒计数"=w294, "定时控制"=w290) -> (w292:T5)
          }
          event "陀螺幅值", "陀螺频率", "加表幅值", "加表频率": Value Change {
            n148 = event-data() -> ()  [unwired: 1 in, 6 out]
            n149 = Reciprocal(x="陀螺频率") -> (1/x=w319:dbl)
            n150 = Multiply(x=w319, y=100.0) -> (x*y=w309:dbl)
            n151 = Round To Nearest(number=w309) -> (nearest integer value=w307:dbl)
            n152 = Bundle By Name(cluster=cluster{"Fs":dbl, "#s":dbl} {"Fs"=1000.0, "#s"=1000.0} ("sampling info"), "Fs"=100.0, "#s"=w307) -> (w314:cluster{"Fs":dbl, "#s":dbl})
            n153 = call <vilib>:"Sine Waveform.vi"("sampling info"=w314, "amplitude"="陀螺幅值", "frequency"="陀螺频率") -> ("signal out"=w332:waveform(dbl))  [unwired: 7 in, 1 out]
            n154 = Reciprocal(x="加表频率") -> (1/x=w325:dbl)
            n155 = Multiply(x=w325, y=100.0) -> (x*y=w310:dbl)
            n156 = Unbundle By Name(w332) -> ("Y"=w328:dbl[])
            n157 = Round To Nearest(number=w310) -> (nearest integer value=w308:dbl)
            n158 = Bundle By Name(cluster=cluster{"Fs":dbl, "#s":dbl} {"Fs"=1000.0, "#s"=1000.0} ("sampling info"), "Fs"=100.0, "#s"=w308) -> (w320:cluster{"Fs":dbl, "#s":dbl})
            n159 = call <vilib>:"Sine Waveform.vi"("sampling info"=w320, "amplitude"="加表幅值", "frequency"="加表频率") -> ("signal out"=w331:waveform(dbl))  [unwired: 7 in, 1 out]
            n160 = Unbundle By Name(w331) -> ("Y"=w329:dbl[])
            n161 = Bundle By Name(cluster=cluster{"陀螺":dbl[], "加表":dbl[]} {"陀螺"=[], "加表"=[]} ("输入簇"), "陀螺"=w328, "加表"=w329) -> (w335:cluster{"陀螺":dbl[], "加表":dbl[]})
            n162 = call <vilib>:"Write.vi"("Register name"="DiJian_data", "Register value"=w335, "Error in"=w333) -> ("Error out"=w334:errorcluster)  [unwired: 10 in, 2 out]
            n163 = call <vilib>:"Write.vi"("Register name"="A_sam_num", "Register value"=w308) -> ("Error out"=w311:errorcluster)  [unwired: 11 in, 2 out]
            n164 = call <vilib>:"Write.vi"("Register name"="G_sam_num", "Register value"=w307, "Error in"=w311) -> ()  [unwired: 10 in, 3 out]
          }
          event "加计大小量程": Value Change {
            n165 = event-data() -> ("NewVal"=w345:enum32{"小量程", "大量程"})  [unwired: 1 in, 5 out]
            n166 = case shown="\"小量程\", 默认" w345 {
              tunnel: [FALSE TRUE] -> w343
              frame "小量程", Default {
              }
              frame "大量程" {
              }
            }
            n167 = call <vilib>:"Write.vi"("Register name"="A_scale", "Register value"=w343, "Error in"=w342) -> ("Error out"=w341:errorcluster)  [unwired: 10 in, 2 out]
          }
        }
      }
      frame "---------- Core ----------" {
        # "Do not put any code in this frame.\n(it is a separator no-op)"
        n168 = call <vilib>:"Add State(s) to Queue__jki_lib_state_machine.vi"("State(s) in (\"\")"=w351) -> ("States Out"=w350:string)  [unwired: 14 in]
      }
      frame Default {
        w361 = 42 items=["No error", "Argument error", "Memory is full", "Out of zone", "End of file", "File already open", "Generic file I/O error", "File not found", "File permission error", "Disk is full", "Duplicate path", "Too many files open", "System feature not enabled", "Resource file not found", "Cannot add resource", "Resource not found", "Image not found", "Image memory error", "Pen does not exist", "Config type invalid", "Config token not found", "Config parse error", "Config memory error", "Bad external code format", "Bad external code offset", "External code not present", "Null window", "Destroy window error", "Null menu", "Print aborted", "Bad print record", "Print driver error", "Windows error during printing", "Memory error during printing", "Print dialog error", "Generic print error", "Invalid device refnum", "Device not found", "Device parameter error", "Device unit error", "Cannot open device", "Device call aborted", "Generic error", "Cancelled by user", "Object ID too low", "Object ID too high", "Object not in heap", "Unknown heap", "Unknown object (invalid DefProc)", "Unknown object (DefProc not in table)", "Message out of range", "Invalid (null) method", "Unknown message", "Manager call not supported", "Bad address", "Network operation in progress", "Network operation timed out", "Connection is busy", "Network attribute not supported", "Network error", "Address in use", "System out of memory", "Connection aborted", "Connection refused", "Not connected", "Already connected", "Connection closed", "Initialization error (interapplication manager)", "Bad occurrence", "Wait on unbound occurrence handler", "Occurrence queue overflow", "Datalog type conflict", "Unused", "Unrecognized type (interapplication manager)", "Memory corrupt", "Failed to make temporary DLL", "Old CIN version", "Drag socket not found", "Failed to load drop-object", "Failed to register OLE object", "Failed to release OLE object", "Format specifier type mismatch", "Unknown format specifier", "Too few format specifiers", "Too many format specifiers", "Scan failed", "Newer CIN version", "Error converting to variant", "Runtime menu error", "Password tampered", "Variant attribute not found", "Incompatible variant data type", "Event data is not available", "Event Store is not present", "Occurrence is not found", "Event Queue is not created", "Event info is not available", "Refnum passed is NULL", "Error retrieving Class GUID", "Error retrieving CoClass GUID", "Error retrieving TypeLib GUID.", "Bad built application magic bytes.", "Specific driver is different from the specific driver associated with the Logical Name.", "There is no session opened to the class driver.", "Max Error", "MAX - Error with config objects", "MAX - Error loading configuration", "MAX - Group not supported"]
        # "Current State"
        # "Do not delete, rename, or modify this frame.\n(this is used to capture unhandled states and typos)"
        # "Handle mistyped state name (developer tool)"
        n169 = Format Into String(format string="Software Exception: Unhandled State \"%s\"." ("message"), error in=w357, w352) -> (resulting string=w360:string, error out=w359:errorcluster)  [unwired: 1 in]
        n170 = call <vilib>:"Error Cluster From Error Code.vi"("show call chain? (False)"=TRUE, "error in (no error)"=w359, "error message (\"\")"=w360, "error code (0)"=w361) -> ("error out"=w358:errorcluster)  [unwired: 5 in]
        n171 = call <vilib>:"Add State(s) to Queue__jki_lib_state_machine.vi"("State(s) in (\"\")"=w356) -> ("States Out"=w355:string)  [unwired: 14 in]
      }
      frame "Initialize Core Data" {
        # "Do not delete, rename, or modify this frame.\n(this is used to determine panel behavior on exit)"
        # "originally closed?"
        # "exe?"
        # "If panel starts closed or is an EXE, then close it when we exit"
        n172 = property class="VI"() -> ("Front Panel.Open"=w370:bool)  [unwired: 2 in, 2 out]
        n173 = property class="App"() -> ("App.Kind"=w369:T3)  [unwired: 2 in, 2 out]
        n174 = control-ref of="Current VI Reference"() -> (w363:refnum<vi>)
        n175 = Not(x=w370) -> (.not. x?=w367:bool)
        n176 = Equal?(x=w369, y=T3."Run Time System" ("Application:Kind")) -> (x = y?=w366:bool)
        n177 = Or(x=w367, y=w366) -> (x .or. y?=w364:bool)
        n178 = Bundle By Name(cluster=w365, "Core.Current VI Reference"=w363, "Core.Close Panel on Exit?"=w364) -> (w372:T5)
        n179 = call <vilib>:"Add State(s) to Queue__jki_lib_state_machine.vi"("State(s) in (\"\")"=w374) -> ("States Out"=w373:string)  [unwired: 14 in]
      }
      frame "Error Handler" {
        # "Unhandled Error -- Display it"
        # "Handle any errors here.\nYou can also output any states to clean-up after errors occur"
        # "Clear error"
        n180 = call <vilib>:"General Error Handler.vi"("error in (no error)"=w376) -> ()  [unwired: 10 in, 5 out]
        n181 = call <vilib>:"Add State(s) to Queue__jki_lib_state_machine.vi"("State(s) in Front (\"\")"="/* Post Error States", "State(s) in (\"\")"=w380) -> ("States Out"=w379:string)  [unwired: 13 in]
      }
      frame "Exit" {
        n182 = call <vilib>:"Add State(s) to Queue__jki_lib_state_machine.vi"("State(s) in (\"\")"=w385) -> ("States Out"=w384:string)  [unwired: 14 in]
      }
      frame "---------- Data ----------" {
        # "Do not put any code in this frame.\n(It is a separator no-op. You can make a copy of this frame to create a new Data frame)"
        n183 = call <vilib>:"Add State(s) to Queue__jki_lib_state_machine.vi"("State(s) in (\"\")"=w389) -> ("States Out"=w388:string)  [unwired: 14 in]
      }
      frame "Data: Initialize" {
        w392 = FALSE  # 定时控制
        w393 = i64 0  # 起始时间
        w394 = i64 0  # 秒计数
        w391 = FALSE
        w397 = u16 0  # 备份控制指令
        w398 = u16 0  # 主份控制指令
        w400 = T6 {" 数据帧名称"="", " 数据"="", "备用操作符"=TRUE, "起始地址"=0, "读写标志"=0, "长度"=0}  # 信息帧
        w401 = T7 {"Current VI Reference"=refnum, "Close Panel on Exit?"=FALSE}  # Core
        n184 = property on="地检按钮" class="Bool (严格)"("Value"=w391) -> ()  [unwired: 2 in, 2 out]
        n185 = call <vilib>:"Write.vi"("Register name"="Zhufen_on", "Register value"=w391) -> ()  [unwired: 11 in, 3 out]
        n186 = Bundle("Core"=w401, "传递队列输入"=w399, "信息帧"=w400, "主份控制指令"=w398, "备份控制指令"=w397, "notifier"=w395, "秒计数"=w394, "起始时间"=w393, "定时控制"=w392) -> (w403:T5)  [unwired: 1 in]
        n187 = call <vilib>:"Add State(s) to Queue__jki_lib_state_machine.vi"("State(s) in (\"\")"=w405) -> ("States Out"=w404:string)  [unwired: 14 in]
        n188 = property on="加计大小量程" class="RadioBtnsControl (严格)"("Value"=enum32{"小量程", "大量程"}."小量程" ("加计大小量程")) -> ()  [unwired: 2 in, 2 out]
      }
      frame "Data: Cleanup" {
        # "Cleanup any data and references, here.\n(this is called automatically, by the Macro: Exit)"
        n189 = Unbundle By Name(w406) -> ("Core.Current VI Reference"=w409:refnum<vi>)
        n190 = Close Reference(reference=w409, error in (no error)=w408) -> (error out=w407:errorcluster)
        n191 = call <vilib>:"Add State(s) to Queue__jki_lib_state_machine.vi"("State(s) in (\"\")"=w411) -> ("States Out"=w410:string)  [unwired: 14 in]
      }
      frame "---------- UI ----------" {
        # "Do not put any code in this frame.\n(It is a separator no-op. You can make a copy of this frame to create a new UI frame)"
        n192 = call <vilib>:"Add State(s) to Queue__jki_lib_state_machine.vi"("State(s) in (\"\")"=w415) -> ("States Out"=w414:string)  [unwired: 14 in]
      }
      frame "UI: Initialize" {
        w417 = u32 0
        # "Initialize the User Interface, here.\n(this is called automatically, by the Macro: Init)"
        n193 = property on="开始测量" class="Bool (严格)"("DisabledEnum"=T2."Enabled" ("禁用")) -> ()  [unwired: 2 in, 2 out]
        n194 = property on="停止测量" class="Bool (严格)"("DisabledEnum"=T2."Disabled and Grayed Out" ("禁用")) -> ()  [unwired: 2 in, 2 out]
        n195 = call <vilib>:"Write.vi"("Register name"="Packs_err_num", "Register value"=w417) -> ()  [unwired: 11 in, 3 out]
        n196 = property on="正确帧计数" class="DigNum (严格)"("Value"=u16 0 ("脉冲  累计")) -> ()  [unwired: 2 in, 2 out]
        n197 = property on="错误帧计数" class="DigNum (严格)"("Value"=w417) -> ()  [unwired: 2 in, 2 out]
        n198 = call <vilib>:"Add State(s) to Queue__jki_lib_state_machine.vi"("State(s) in (\"\")"=w424) -> ("States Out"=w423:string)  [unwired: 14 in]
      }
      frame "UI: Cursor Set" {
        # "Argument"
        # "Set and Unset Cursor Busy.\n(Usage: \"UI: Cursor Set >> Busy|Idle\")"
        n199 = case shown="\"Idle\", 默认" w425 {
          tunnel: w427 -> [w432 w434]
          tunnel: [w431 w433] -> w426
          frame "Idle", Default {
            n200 = call <vilib>:"Unset Busy.vi"("error in (no error)"=w432) -> ("error out"=w431:errorcluster)  [unwired: 10 in]
          }
          frame "Busy" {
            n201 = call <vilib>:"Set Busy.vi"("error in (no error)"=w434) -> ("error out"=w433:errorcluster)  [unwired: 9 in, 1 out]
          }
        }
        n202 = call <vilib>:"Add State(s) to Queue__jki_lib_state_machine.vi"("State(s) in (\"\")"=w430) -> ("States Out"=w429:string)  [unwired: 14 in]
      }
      frame "UI: Front Panel State" {
        # "Set Front Panel Open or Closed\n(Usage: \"UI: Front Panel State >> Open|Close\")"
        n203 = disable-structure shown="启用" {
          disable-tunnel: w438 -> [w445 w468]
          disable-tunnel: [w444 w468] -> w437
          disable-tunnel: w436 -> [w443 _]
          disable-tunnel: w435 -> [w441 _]
          frame Disabled {
            # "Argument"
            n204 = Unbundle By Name(w443) -> ("Core.Current VI Reference"=w442:refnum<vi>)
            n205 = case shown="\"Open\", 默认" w441 {
              tunnel: w445 -> [w449 w462]
              tunnel: [w451 w463] -> w444
              tunnel: w442 -> [w450 w460]
              frame "Open", Default {
                n206 = property class="VI"(reference=w450, error in=w449) -> (reference out=w447:refnum<vi>, error out=w448:errorcluster, "Front Panel.Open"=w446:bool)
                n207 = case shown="假" w446 {
                  tunnel: [w454 w457] -> w451
                  tunnel: w448 -> [w453 w457]
                  tunnel: w447 -> [w452 _]
                  frame False {
                    n208 = invoke class="VI" method="FP.Open"(reference=w452, error in=w453, "Activate"=TRUE, "State"=T4."Standard") -> (error out=w454:errorcluster)  [unwired: 1 in, 4 out]
                  }
                  frame True {
                  }
                }
              }
              frame "Close" {
                n209 = property class="VI"(reference=w460, error in=w462) -> (reference out=w459:refnum<vi>, error out=w461:errorcluster, "Front Panel.Open"=w458:bool)
                n210 = case shown="真" w458 {
                  tunnel: [w464 w467] -> w463
                  tunnel: w461 -> [w464 w466]
                  tunnel: w459 -> [_ w465]
                  frame False {
                  }
                  frame True {
                    n211 = invoke class="VI" method="FP.Close"(reference=w465, error in=w466) -> (error out=w467:errorcluster)  [unwired: 1 in, 2 out]
                  }
                }
              }
            }
          }
          frame Enabled {
          }
        }
        n212 = call <vilib>:"Add State(s) to Queue__jki_lib_state_machine.vi"("State(s) in (\"\")"=w440) -> ("States Out"=w439:string)  [unwired: 14 in]
      }
      frame "---------- Macro ----------" {
        # "Do not put any code in this frame.\n(It is a separator no-op. You can make a copy of this frame to create a new Macro frame)"
        n213 = call <vilib>:"Add State(s) to Queue__jki_lib_state_machine.vi"("State(s) in (\"\")"=w472) -> ("States Out"=w471:string)  [unwired: 14 in]
      }
      frame "Macro: Initialize" {
        w473 = "Data: Initialize\nInitialize Core Data\nUI: Initialize\nUI: Front Panel State >> Open"  # Data: Initialize Initialize Core Data UI: Initialize UI: Front Panel State >> Open
        # "Initialization Macro\n(This is called once, when the VI starts)"
        n214 = call <vilib>:"Add State(s) to Queue__jki_lib_state_machine.vi"("State(s) in Front (\"\")"=w473, "State(s) in (\"\")"=w477) -> ("States Out"=w476:string)  [unwired: 13 in]
      }
      frame "Macro: Exit" {
        # "Exit Macro\n(This is called once, when the VI exits)"
        n215 = Unbundle By Name(w484) -> ("Core.Close Panel on Exit?"=w483:bool)
        n216 = Select(t="UI: Front Panel State >> Close", s=w483, f="") -> (s? t:f=w480:string)
        n217 = call <vilib>:"Add State(s) to Queue__jki_lib_state_machine.vi"("State(s) in (\"\")"=w480, "State(s) at Back (\"\")"="Data: Cleanup\nExit") -> ("States Out"=w478:string)  [unwired: 13 in]
        n218 = call <vilib>:"Add State(s) to Queue__jki_lib_state_machine.vi"("State(s) in Front (\"\")"=w478, "State(s) in (\"\")"=w487) -> ("States Out"=w486:string)  [unwired: 13 in]
      }
      frame "----------Request----------" {
        # "Template Separator\n(You can make a copy of, or modify, this frame)"
        n219 = call <vilib>:"Add State(s) to Queue__jki_lib_state_machine.vi"("State(s) in (\"\")"=w491) -> ("States Out"=w490:string)  [unwired: 14 in]
      }
      frame "Request:Write" {
        n220 = in-place {
          in-place-border: w495 -> [w501]
          in-place-border: [w500] -> w494
          in-place-border: w492 -> [w499]
          n221 = in-place-cluster #1(w496) -> ("传递队列输入"=w505:refnum<queue>, "信息帧"=w504:T6)
          n222 = in-place {
            in-place-border: w499 -> [w506]
            n223 = in-place-cluster #2(w504) -> ("数据"=w511:string)  [unwired: 5 out]
            n224 = in-place-cluster #2("数据帧名称"=w506, "数据"=w511, "备用操作符"=TRUE, "起始地址"=0, "读写标志"=1, "长度"=0) -> (w503:T6)
          }
          n225 = Enqueue Element(queue=w505, element=w503, error in (no error)=w501) -> (queue out=w502:refnum<queue>, error out=w500:errorcluster)  [unwired: 1 in, 1 out]
          n226 = in-place-cluster #1("传递队列输入"=w502, "信息帧"=w503) -> (w493:T5)
        }
        n227 = call <vilib>:"Add State(s) to Queue__jki_lib_state_machine.vi"("State(s) in (\"\")"=w498) -> ("States Out"=w497:string)  [unwired: 14 in]
      }
      frame "Config:Write" {
        n228 = in-place {
          in-place-border: w515 -> [w521]
          in-place-border: [w520] -> w514
          in-place-border: w512 -> [w519]
          n229 = in-place-cluster #3(w516) -> ("传递队列输入"=w525:refnum<queue>, "信息帧"=w524:T6)
          n230 = in-place {
            in-place-border: w519 -> [w526]
            n231 = in-place-cluster #4(w524) -> ("数据"=w531:string)  [unwired: 5 out]
            n232 = in-place-cluster #4("数据帧名称"=w526, "数据"=w531, "备用操作符"=TRUE, "起始地址"=0, "读写标志"=2, "长度"=0) -> (w523:T6)
          }
          n233 = Enqueue Element(queue=w525, element=w523, error in (no error)=w521) -> (queue out=w522:refnum<queue>, error out=w520:errorcluster)  [unwired: 1 in, 1 out]
          n234 = in-place-cluster #3("传递队列输入"=w522, "信息帧"=w523) -> (w513:T5)
        }
        n235 = call <vilib>:"Add State(s) to Queue__jki_lib_state_machine.vi"("State(s) in (\"\")"=w518) -> ("States Out"=w517:string)  [unwired: 14 in]
      }
      frame "Request:OPEN1553B" {
        n236 = in-place {
          in-place-border: w535 -> [w542]
          in-place-border: [w541] -> w534
          in-place-border: w532 -> [w539]
          n237 = in-place-cluster #5(w536) -> ("传递队列输入"=w545:refnum<queue>, "信息帧"=w540:T6)
          n238 = in-place {
            in-place-border: w539 -> [w546]
            n239 = in-place-cluster #6(w540) -> ()  [unwired: 6 out]
            n240 = in-place-cluster #6("数据帧名称"=w546, "数据"="$B\n", "备用操作符"=TRUE, "起始地址"=0, "读写标志"=1, "长度"=0) -> (w544:T6)
          }
          n241 = Enqueue Element(queue=w545, element=w544, error in (no error)=w542) -> (queue out=w543:refnum<queue>, error out=w541:errorcluster)  [unwired: 1 in, 1 out]
          n242 = in-place-cluster #5("传递队列输入"=w543, "信息帧"=w540) -> (w533:T5)
        }
        n243 = call <vilib>:"Add State(s) to Queue__jki_lib_state_machine.vi"("State(s) in (\"\")"=w538) -> ("States Out"=w537:string)  [unwired: 14 in]
      }
      frame "Request:Close1553B" {
        n244 = in-place {
          in-place-border: w554 -> [w563]
          in-place-border: [w562] -> w553
          n245 = in-place-cluster #7(w555) -> ("传递队列输入"=w565:refnum<queue>, "信息帧"=w559:T6)
          n246 = in-place {
            n247 = in-place-cluster #8(w559) -> ()  [unwired: 6 out]
            n248 = in-place-cluster #8("数据帧名称"="1553B_CMD", "数据"="$", "备用操作符"=TRUE, "起始地址"=0, "读写标志"=1, "长度"=0) -> (w564:T6)
          }
          n249 = in-place {
            n250 = in-place-cluster #9(w559) -> ()  [unwired: 6 out]
            n251 = in-place-cluster #9("数据帧名称"="1553B_CMD", "数据"="$Z\n", "备用操作符"=TRUE, "起始地址"=0, "读写标志"=1, "长度"=0) -> (w560:T6)
          }
          n252 = Enqueue Element(queue=w565, element=w564, error in (no error)=w563) -> (queue out=w561:refnum<queue>, error out=w562:errorcluster)  [unwired: 1 in, 1 out]
          n253 = Enqueue Element(queue=w561, element=w560) -> (queue out=w558:refnum<queue>)  [unwired: 2 in, 2 out]
          n254 = in-place-cluster #7("传递队列输入"=w558, "信息帧"=w559) -> (w552:T5)
        }
        n255 = call <vilib>:"Add State(s) to Queue__jki_lib_state_machine.vi"("State(s) in (\"\")"=w557) -> ("States Out"=w556:string)  [unwired: 14 in]
      }
      frame "Request:Read" {
        n256 = in-place {
          in-place-border: w580 -> [w585]
          in-place-border: [w584] -> w579
          n257 = in-place-cluster #10(w581) -> ("传递队列输入"=w589:refnum<queue>, "信息帧"=w588:T6)
          n258 = in-place {
            n259 = in-place-cluster #11(w588) -> ("数据"=w594:string)  [unwired: 5 out]
            n260 = in-place-cluster #11("数据帧名称"="GNSS1", "数据"=w594, "备用操作符"=TRUE, "起始地址"=0, "读写标志"=0, "长度"=0) -> (w587:T6)
          }
          n261 = Enqueue Element(queue=w589, element=w587, error in (no error)=w585) -> (queue out=w586:refnum<queue>, error out=w584:errorcluster)  [unwired: 1 in, 1 out]
          n262 = in-place-cluster #10("传递队列输入"=w586, "信息帧"=w587) -> (w578:T5)
        }
        n263 = call <vilib>:"Add State(s) to Queue__jki_lib_state_machine.vi"("State(s) in (\"\")"=w583) -> ("States Out"=w582:string)  [unwired: 14 in]
      }
      frame "----------Usr----------" {
        # "Template Separator\n(You can make a copy of, or modify, this frame)"
        n264 = call <vilib>:"Add State(s) to Queue__jki_lib_state_machine.vi"("State(s) in (\"\")"=w599) -> ("States Out"=w598:string)  [unwired: 14 in]
      }
      frame "Exit:all" {
        n265 = call <vilib>:"Add State(s) to Queue__jki_lib_state_machine.vi"("State(s) in Front (\"\")"="Macro: Exit", "State(s) in (\"\")"=w604) -> ("States Out"=w603:string)  [unwired: 13 in]
      }
      frame "Usr:Frame-init" {
        n266 = in-place {
          n267 = in-place-cluster #12(w606) -> ()  [unwired: 1 out]
          n268 = Initialize Array(u8 0 ("元素"), 218 ("维数大小")) -> (w613:u8[])
          n269 = Replace Array Subset(array=w613, new element=u8[] [170, 85, 218, 0], index=0 ("索引")) -> (w610:u8[])
          n270 = Byte Array To String(unsigned byte array=w610) -> (string=w616:string)
          n271 = in-place-cluster #12("信息帧.数据"=w616) -> (w605:T5)
        }
        n272 = call <vilib>:"Add State(s) to Queue__jki_lib_state_machine.vi"("State(s) in (\"\")"=w609) -> ("States Out"=w608:string)  [unwired: 14 in]
      }
      frame "Usr:Frame-set" {
        n273 = disable-structure shown="禁用" {
          disable-tunnel: ["Request:Write" ("State(s) in Front (\"\")") _] -> w618
          frame Disabled {
          }
          frame Enabled {
          }
        }
        n274 = call <vilib>:"Add State(s) to Queue__jki_lib_state_machine.vi"("State(s) in (\"\")"=w621, "State(s) at Back (\"\")"=w618) -> ("States Out"=w620:string)  [unwired: 13 in]
      }
      frame "Usr:Update_timestap" {
        n275 = Get Date/Time In Seconds() -> (seconds since 1Jan1904=w637:timestamp)
        n276 = Seconds To Date/Time(time stamp (now)=w637) -> (date time rec=w629:T1)  [unwired: 1 in]
        n277 = Unbundle By Name(w629) -> ("时"=w630:i32, "分"=w633:i32, "秒"=w623:i32)
        n278 = Multiply(x=w630, y=60) -> (x*y=w632:i32)
        n279 = Add(x=w632, y=w633) -> (x+y=w634:i32)
        n280 = Multiply(x=w634, y=60) -> (x*y=w636:i32)
        n281 = Add(x=w636, y=w623) -> (x+y=w628:i32)
        n282 = To Quad Integer(1:w628) -> (0:w627:i64)
        n283 = call <vilib>:"Add State(s) to Queue__jki_lib_state_machine.vi"("State(s) in (\"\")"=w639) -> ("States Out"=w638:string)  [unwired: 14 in]
        n284 = Bundle By Name(cluster=w626, "起始时间"=w627) -> (w625:T5)
      }
    }
  }
  n285 = while {
    tunnel: "notifier" -> [w645]
    stop <- w644 stop-if-true
    n286 = call "stop_message.vi"("notifier"=w645) -> ("Exit？"=w644:bool)  [unwired: 9 in, 1 out]
    n287 = call <vilib>:"Read.vi"("Register name"="Zhufen_on") -> ("Register value"=w642:variant)  [unwired: 11 in, 3 out]
    n288 = call-poly <vilib>:"Convert.vi"("Register value in"=w642) -> ("Register value out"=w641:bool)  [unwired: 13 in, 1 out]
    n289 = Wait (ms)(milliseconds to wait=u32 100 ("等待时间（毫秒）")) -> ()  [unwired: 1 out]
    n290 = case shown="真" w641 {
      frame False {
      }
      frame True {
        n291 = call <vilib>:"Read.vi"("Register name"="Packs_err_num") -> ("Register value"=w649:variant)  [unwired: 11 in, 3 out]
        n292 = call <vilib>:"Read.vi"("Register name"="Run_mode") -> ("Register value"=w655:variant)  [unwired: 11 in, 3 out]
        n293 = call-poly <vilib>:"Convert.vi"("Register value in"=w649) -> ("Register value out"=→"错误帧计数":u32)  [unwired: 13 in, 1 out]
        n294 = call-poly <vilib>:"Convert.vi"("Register value in"=w655) -> ("Register value out"=w653:u8)  [unwired: 13 in, 1 out]
        n295 = call <vilib>:"Read.vi"("Register name"="Packs_ok_num") -> ("Register value"=w648:variant)  [unwired: 11 in, 3 out]
        n296 = call-poly <vilib>:"Convert.vi"("Register value in"=w648) -> ("Register value out"=→"正确帧计数":u32)  [unwired: 13 in, 1 out]
        n297 = call <vilib>:"Read.vi"("Timeout"=1, "Register name"="1553BZhuFenRecv_stat") -> ("Register value"=w656:variant, "Register value read?"=w652:bool)  [unwired: 10 in, 2 out]
        n298 = case shown="真" w652 {
          tunnel: w656 -> [_ w668]
          tunnel: w653 -> [_ w667]
          frame False {
          }
          frame True {
            n299 = call "state_sep.vi"("Register value"=w668, "MODE"=w667) -> ("G1陀螺脉冲数"=→"主份G1陀螺脉冲数":dbl, "G2陀螺脉冲数"=→"主份G2陀螺脉冲数":dbl, "G3陀螺脉冲数"=→"主份G3陀螺脉冲计数":dbl, "A1加速度计脉冲数"=→"主份A1加速度计脉冲计数":dbl, "A2加速度计脉冲数"=→"主份A2加速度计脉冲计数":dbl, "温度"=→"温度":string, "脉冲计数"=→"脉冲计数":string, "A3加速度计脉冲数"=→"主份A3加速度计脉冲计数":dbl)  [unwired: 17 in, 1 out]
          }
        }
      }
    }
  }
